vi "Optics_GetStatus.VI"(6 "Error in":errorcluster, 8 "Motor":dbl, 9 "VISA":refnum<visa-resource-name>) -> (0 "Error out":errorcluster, 1 "Moving":bool, 2 "Velocity":dbl, 3 "Position":dbl)   [LabVIEW 2021]
panel:
  out "String read":string
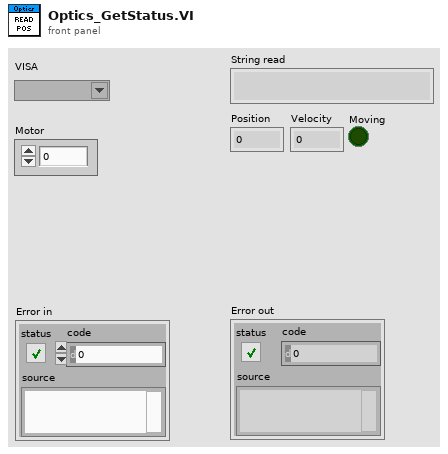
[diagram p1: front panel]
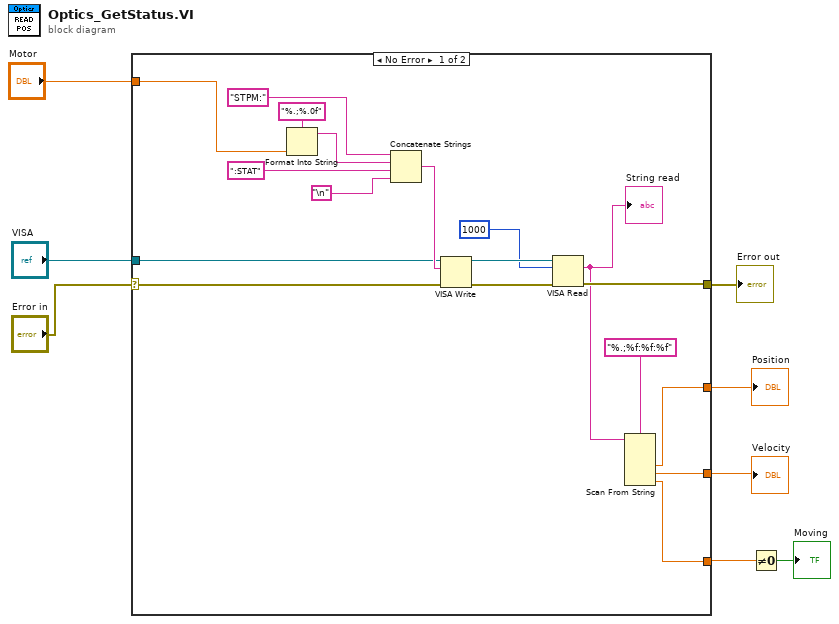
[diagram p0: block diagram]
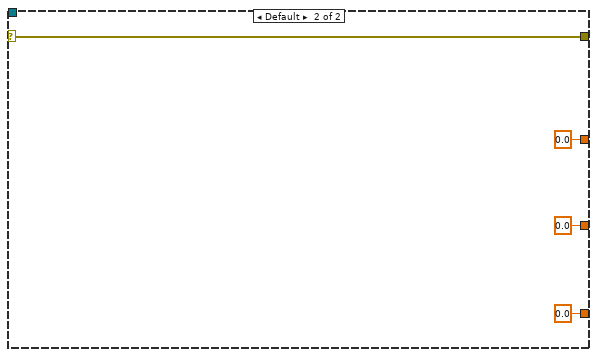
[diagram p2: hidden frame]
diagram:
  n1 = case shown="No Error" "Error in" {
    selector: "Error in" -> [w16 w30]
    tunnel: [w14 w30] -> w8
    tunnel: "Motor" -> [w23 _]
    tunnel: "VISA" -> [w15 _]
    tunnel: [w11 0.0] -> w2
    tunnel: [w10 0.0] -> w4
    tunnel: [w9 0.0] -> w3
    frame No Error {
      n2 = Format Into String(format string="%.;%.0f", w23) -> (resulting string=w26:string)  [unwired: 2 in, 1 out]
      n3 = Concatenate Strings("STPM:", w26, ":STAT", "\n") -> (w21:string)
      n4 = VISA Write(VISA resource name=w15, write buffer=w21, error in (no error)=w16) -> (VISA resource name out=w20:refnum<visa-resource-name>, error out=w17:errorcluster)  [unwired: 1 out]
      n5 = VISA Read(VISA resource name=w20, byte count=u32 1000, error in (no error)=w17) -> (read buffer=w12:string, error out=w14:errorcluster)  [unwired: 2 out]
      "String read" <- w12
      n6 = Scan From String(format string="%.;%f:%f:%f", input string=w12) -> (output 1=w9:dbl, output 2=w10:dbl, output 3=w11:dbl)  [unwired: 5 in, 3 out]
    }
    frame Default {
    }
  }
  "Error out" <- w8
  "Position" <- w3
  "Velocity" <- w4
  n7 = Not Equal To 0?(x=w2) -> (x != 0?=→"Moving":bool)
